vi "Preset_Edit_Range2txt.vi"(10 "Engineering units":string, 11 "Range":dbl) -> (2 "RangeInfo":string)   [LabVIEW 2020, in "Sgraph_lib_V1.lvlib" / "Gviewer.lvclass"]
doc: "Convert Range & Engineering units to Range info including the -1 (not defined) value"
uses:
  Gviewer.lvclass
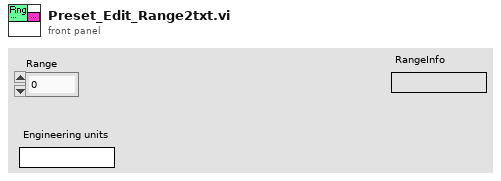
[diagram p1: front panel]
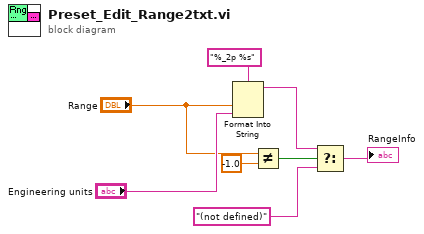
[diagram p0: block diagram]
diagram:
  n1 = Format Into String(format string="%_2p %s", "Range", "Engineering units") -> (resulting string=w3:string)  [unwired: 2 in, 1 out]
  n2 = Not Equal?(x="Range", y=-1.0) -> (x != y?=w4:bool)
  n3 = Select(t=w3, s=w4, f="(not defined)") -> (s? t:f=→"RangeInfo":string)
